vi "Command Data 2 Control Target.vi"(9 "Current Command":dbl[](array[numeric]), 11 "Current Target":T1={"Displacements"=[4.0, 3.0, 0.0, 0.0, 0.0, 0.0], "Command Type"=[enum."<None>", enum."Displacement", enum."<None>", enum."Force", enum."<None>", enum."Force"], "Forces"=[0.0, 0.0, 0.0, 6.0, 0.0, 8.0]}) -> (2 "Output":T1)   [LabVIEW 2009]
uses:
  Target Data.ctl
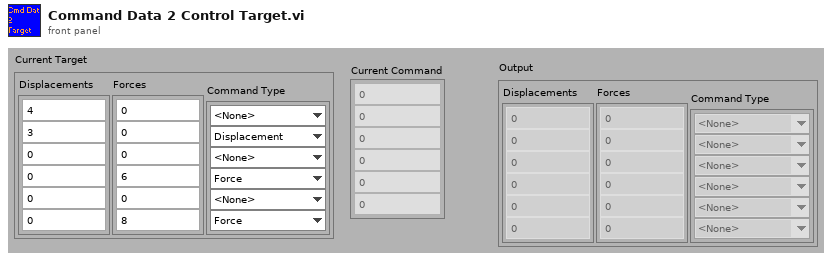
[diagram p1: front panel]
types:
  T1 = typedef "Target Data.ctl" = cluster{"Displacements":dbl[], "Command Type":enum16{"<None>", "Displacement", "Force"}[], "Forces":dbl[]}
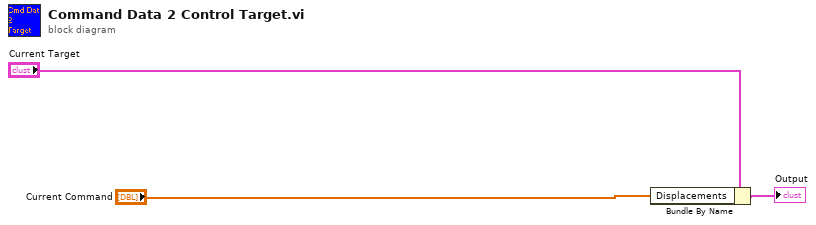
[diagram p0: block diagram]
diagram:
  n1 = Bundle By Name(cluster="Current Target", "Displacements"="Current Command") -> (→"Output":T1)
